vi "Find variables.vi"(11 "XML":string) -> (2 "Variable Clusters out":T1, 3 "Name":string[](array[string]))   [LabVIEW 2012, in "Design Server.lvlib"]
uses:
  Design Server.lvlib
  Variable cluster.ctl
panel:
  out "Eval Regions":string[](array[string])
  out "Name.Sub":string[](array[string])
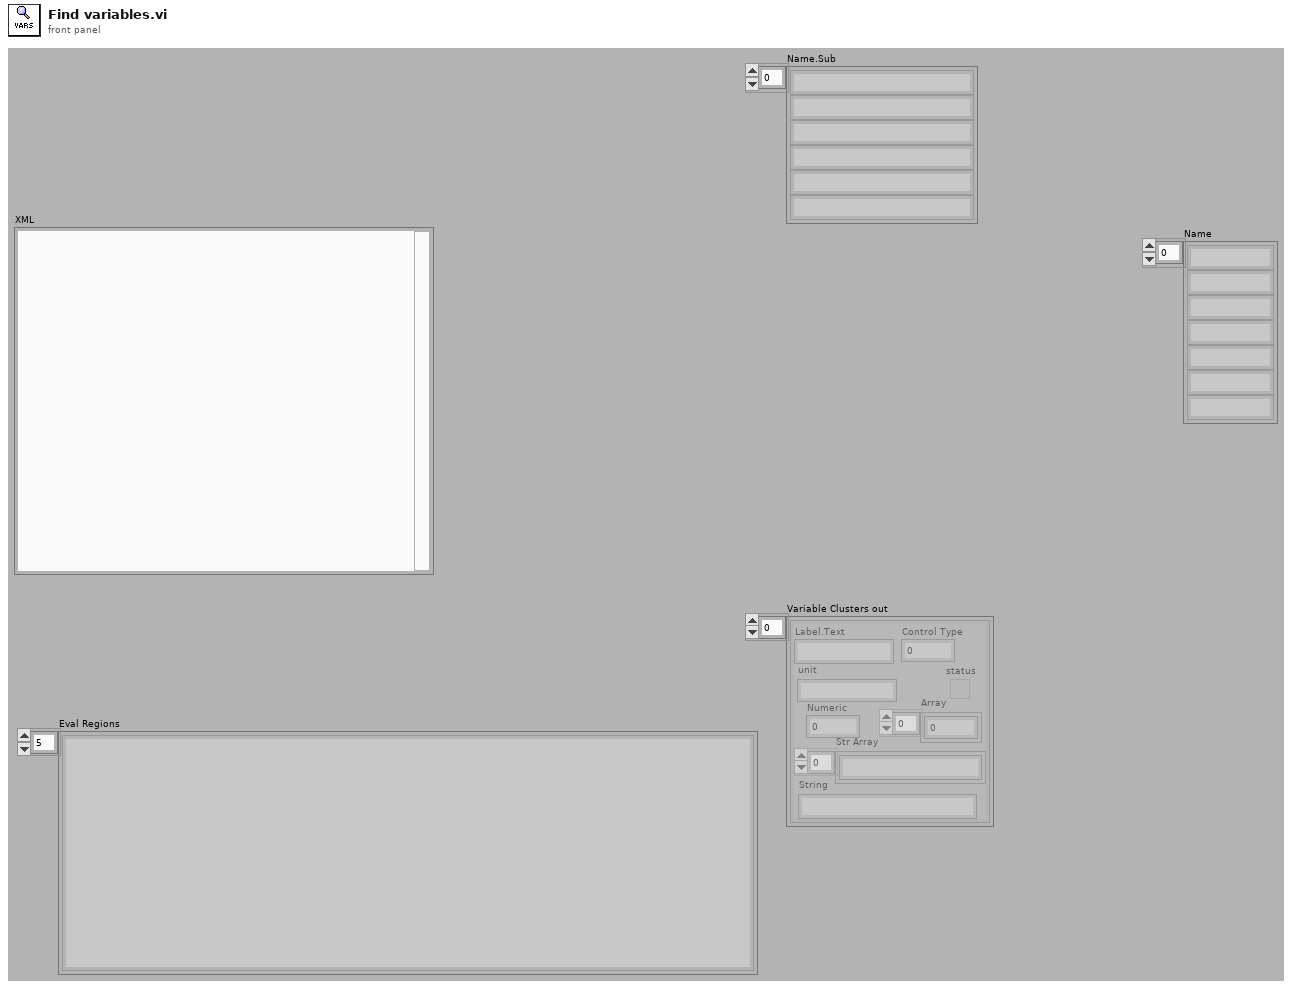
[diagram p1: front panel]
types:
  T1 = typedef "Design Server.lvlib/Variable cluster.ctl" = cluster{"Label.Text":string, "Control Type":u32, "Numeric":dbl, "Array":dbl[], "status":bool, "Str Array":string[], "String":string, "unit":string}[]
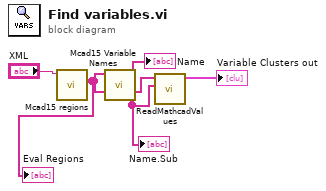
[diagram p0: block diagram]
diagram:
  n1 = call "Mcad15 regions.vi"("file text in"="XML") -> ("Eval Regions"=w3:string[])  [unwired: 9 in, 1 out]
  "Eval Regions" <- w3
  n2 = call "Mcad15 Variable Names.vi"("Eval Regions"=w3) -> ("Name"=→"Name":string[], "Name.Sub"=w1:string[])  [unwired: 8 in]
  "Name.Sub" <- w1
  n3 = call "ReadMathcadValues.vi"("Name.Sub"=w1, "Regions"=w3) -> ("Variable Clusters out"=→"Variable Clusters out":T1)  [unwired: 9 in]
